vi "updateColumnHeaders.vi"(8 "error in (no error)":errorcluster, 11 "TestDataLog in":refnum<class "TestDataLog.lvclass">) -> (0 "error out":errorcluster, 3 "TestDataLog out":refnum<class "TestDataLog.lvclass">)   [LabVIEW 2016, in "TestDataLog.lvclass"]
uses:
  TestDataLog.lvclass
  D:/Code/ts_dcabt/Common_Log/Log/Log.lvclass
  Common_Log/Log/Log.lvclass/Log.ctl
  Common_Log/Log/Log.lvclass
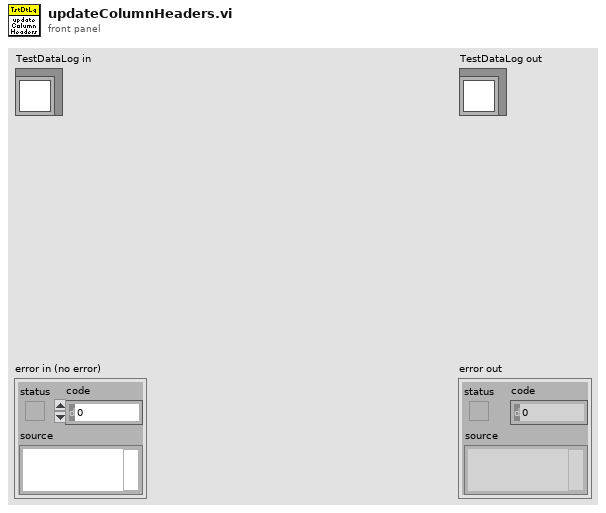
[diagram p1: front panel]
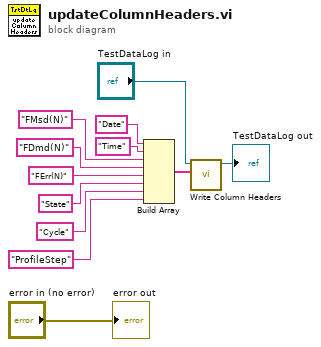
[diagram p0: block diagram]
diagram:
  n1 = Build Array("Date" ("element"), "Time", "FMsd(N)", "FDmd(N)", "FErr(N)", "State", "Cycle", "ProfileStep") -> (w4:string[])
  n2 = call "Write Column Headers.vi"("Column Headers"=w4, "Logger in"="TestDataLog in") -> ("Logger out"=→"TestDataLog out":refnum<class "TestDataLog.lvclass">)  [unwired: 9 in]
  "error out" <- "error in (no error)"
